vi "Build CHM.vi"() -> ()   [LabVIEW 2015]
uses:
  <vilib>/Utility/config.llb/Read Key (String).vi
  <vilib>/Utility/config.llb/Read Key (Path).vi
  Classes/CHM Generator/CHM Generator.lvclass
  <vilib>/Utility/config.llb/NI_LVConfig.lvlib
panel:
  out "standard output":string
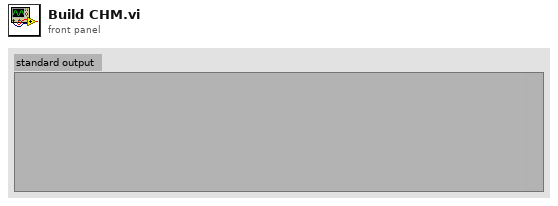
[diagram p1: front panel]
types:
  T1 = typedef "NI_LVConfig.lvlib/Config Data RefNum.ctl" = refnum<k1>
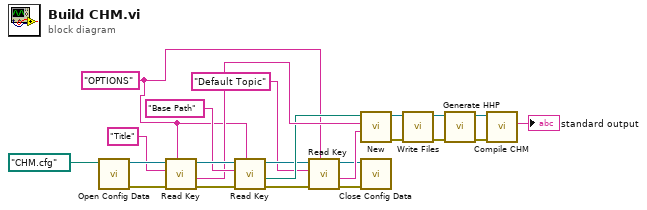
[diagram p0: block diagram]
diagram:
  w1 = "OPTIONS" ("section")
  n1 = call <vilib>:"Open Config Data.vi"("configuration file path"=path "CHM.cfg" ("Path")) -> ("error out"=w14:errorcluster, "refnum"=w15:T1)  [unwired: 8 in, 1 out]
  n2 = call-poly <vilib>:"Read Key.vi"("section"=w1, "error in (no error)"=w14, "key"="Title", "refnum"=w15) -> ("error out"=w12:errorcluster, "value"=w9:string, "refnum out"=w11:T1)  [unwired: 4 in, 1 out]
  n3 = call-poly <vilib>:"Read Key.vi"("section"=w1, "error in (no error)"=w12, "key"="Base Path", "refnum"=w11) -> ("error out"=w8:errorcluster, "value"=w7:path, "refnum out"=w6:T1)  [unwired: 4 in, 1 out]
  n4 = call-poly <vilib>:"Read Key.vi"("section"=w1, "error in (no error)"=w8, "key"="Default Topic", "refnum"=w6) -> ("error out"=w3:errorcluster, "value"=w4:string, "refnum out"=w2:T1)  [unwired: 4 in, 1 out]
  n5 = call "New.vi"("Default topic"=w4, "Title"=w9, "Base Path"=w7) -> ("error out"=w22:errorcluster, "CHM Generator out"=w23:refnum<class "CHM Generator.lvclass">)  [unwired: 7 in]
  n6 = call <vilib>:"Close Config Data.vi"("error in (no error)"=w3, "refnum"=w2) -> ()  [unwired: 8 in, 2 out]
  n7 = call-dynamic "Write Files.vi"("error in (no error)"=w22, "CHM Generator in"=w23) -> ("error out"=w21:errorcluster, "CHM Generator out"=w20:refnum<class "CHM Generator.lvclass">)  [unwired: 8 in]
  n8 = call-dynamic "Generate HHP.vi"("error in (no error)"=w21, "CHM Generator in"=w20) -> ("error out"=w18:errorcluster, "CHM Generator out"=w19:refnum<class "CHM Generator.lvclass">)  [unwired: 8 in]
  n9 = call "Compile CHM.vi"("error in (no error)"=w18, "CHM Generator in"=w19) -> ("standard output"=→"standard output":string)  [unwired: 7 in, 2 out]
